vi "标签打印.vi"(8 "error in (no error)":errorcluster caption="错误输入（无错误）", 11 "barcode":string="C0C01B2473005") -> (0 "error out":errorcluster caption="错误输出", 3 "Print":string)   [LabVIEW 2017]
uses:
  D:/Inspect System/Source Code/Andafa.IO.Helper.dll
  Andafa.IO.Helper.dll
panel:
  in  "accessKey":string="a45b2d3334ffs_"
  in  "Url":string="http://10.6.1.31:8080/MesInnerpackLineIO.asmx"
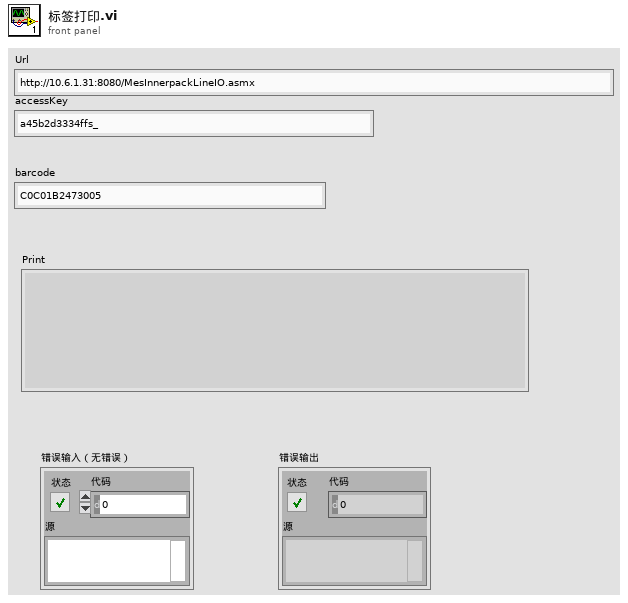
[diagram p1: front panel]
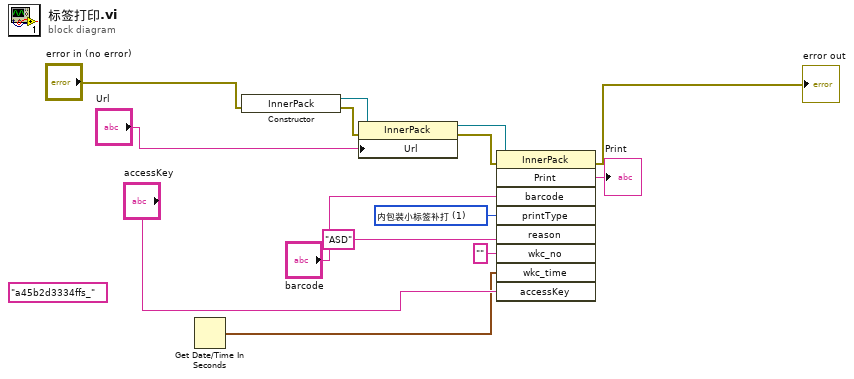
[diagram p0: block diagram]
diagram:
  w5 = 1 items=["内包装小标签打印", "内包装小标签补打"] ("printType")
  (unwired) "a45b2d3334ffs_" ("accessKey")
  n1 = Get Date/Time In Seconds() -> (seconds since 1Jan1904=w2:timestamp)
  n2 = constructor class="InnerPack"(error in="error in (no error)") -> (reference out=w13:refnum<k24>, error out=w9:errorcluster)  [unwired: 2 in, 1 out]
  n3 = property on="属性节点" class="InnerPack"(reference=w13, error in=w9, "Url"="Url") -> (reference out=w12:refnum<k24>, error out=w10:errorcluster)
  n4 = invoke on="调用节点" class="InnerPack" method="Print"(reference=w12, error in=w10, "barcode"="barcode", "printType"=w5, "reason"="ASD", "wkc_no"="", "wkc_time"=w2, "accessKey"="accessKey") -> (error out=→"error out":errorcluster, "Print"=→"Print":string)  [unwired: 1 in, 7 out]
